vi "Set Strings from Ref.vi"(8 "error in (no error)":errorcluster, 9 "Language Index (0)":i32, 10 "GObj Refnum":refnum<vi>, 11 "StringControl in":refnum<class "StringControl.lvclass">) -> (0 "error out":errorcluster, 3 "StringControl out":refnum<class "StringControl.lvclass">)   [LabVIEW 2013, in "SET Project Data.lvlib" / "StringControl.lvclass"]
uses:
  StringControl.lvclass
  Control/Control.lvclass
  GObject/GObject.lvclass
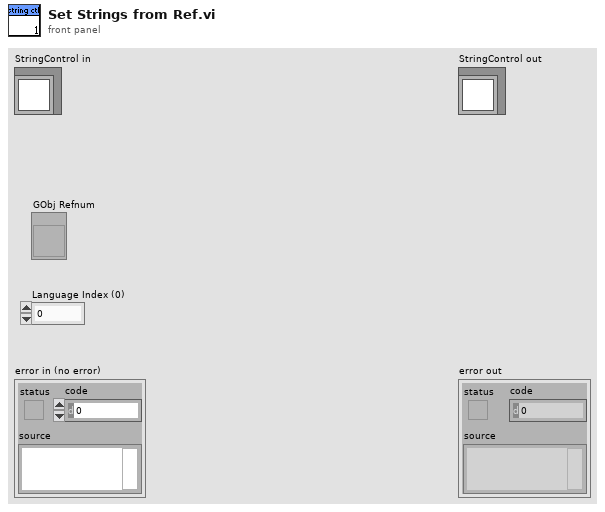
[diagram p1: front panel]
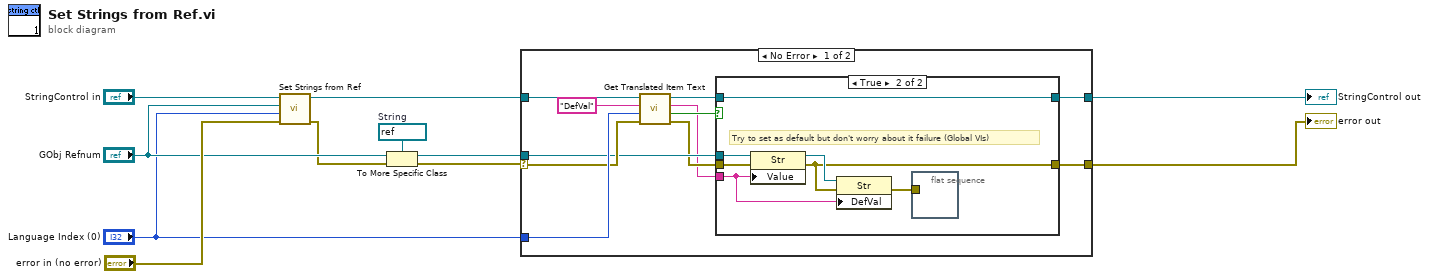
[diagram p0: block diagram]
diagram:
  w9 = refnum<vi> refnum  # String
  n1 = call-parent "Set Strings from Ref.vi"("error in (no error)"="error in (no error)", "Language Index (0)"="Language Index (0)", "GObj Refnum"="GObj Refnum", "Control in"="StringControl in") -> ("error out"=w7:errorcluster, "Control out"=w6:refnum<class "StringControl.lvclass">)  [unwired: 6 in]
  n2 = To More Specific Class(target class=w9, reference="GObj Refnum", error in=w7) -> (specific class reference=w5:refnum<vi>, error out=w4:errorcluster)
  n3 = case shown="No Error" w4 {
    selector: w4 -> [w19 w32]
    tunnel: w5 -> [w17 _]
    tunnel: w6 -> [w21 w33]
    tunnel: "Language Index (0)" -> [w20 _]
    tunnel: [w12 w33] -> w2
    tunnel: [w15 w32] -> w1
    frame No Error {
      n4 = call "Get Translated Item Text.vi"("error in (no error)"=w19, "LangIndex (0)"=w20, "ItemName"="DefVal", "GObject in"=w21) -> ("error out"=w16:errorcluster, "Found?"=w18:bool, "Translated Text (ASCII)"=w14:string, "GObject out"=w13:refnum<class "StringControl.lvclass">)  [unwired: 4 in]
      n5 = case shown="True" w18 {
        tunnel: w17 -> [_ w31]
        tunnel: w14 -> [_ w29]
        tunnel: w16 -> [w24 w27]
        tunnel: [w24 w26] -> w15
        tunnel: w13 -> [w23 w28]
        tunnel: [w23 w28] -> w12
        frame False {
        }
        frame True {
          # "Try to set as default but don't worry about it failure (Global VIs)"
          n6 = property class="Str"(reference=w31, error in=w27, "Value"=w29) -> (reference out=w30:refnum<vi>, error out=w26:errorcluster)
          n7 = property class="Str"(reference=w30, error in=w26, "DefVal"=w29) -> (error out=w25:errorcluster)  [unwired: 1 out]
          n8 = flat-sequence {
            tunnel: w25 -> [_]
            frame #0 {
            }
          }
        }
      }
    }
    frame Error {
    }
  }
  "error out" <- w1
  "StringControl out" <- w2
